vi "routine.vi"() -> ()   [LabVIEW 2011]
panel:
  in  "Boolean":bool
  in  "Filename":path=path "C:/Users/Sinha/Desktop/Ankle/2.csv"
  in  "Target":bool=TRUE
  in  "AI 2":bool
  in  "AI 1":bool=TRUE
  out "?":bool
  in  "AI 0":bool=TRUE
  in  "Target":dbl=0.5 caption="Offset"
  in  "Sample Rate Hz.":dbl=200.0
  out "Waveform Chart":dbl[][](graph)=[[-5.0, -5.0, -5.0, 0.5], [-5.0, -5.0, -5.0, 0.5], [-5.0, -5.0, -5.0, 0.5], [-5.0, -5.0, -5.0, 0.5], [-5.0, -5.0, -5.0, 0.5], [-5.0, -5.0, -5.0, 0.5], [-5.0, -5.0, -5.0, 0.5], [-5.0, -5.0, -5.0, 0.5], [-5.0, -5.0, -5.0, 0.5], [-5.0, -5.0, -5.0, 0.5], [-5.0, -5.0, -5.0, 0.5], [-5.0, -5.0, -5.0, 0.5], [-5.0, -5.0, -5.0, 0.5], [-5.0, -5.0, -5.0, 0.5], [-5.0, -5.0, -5.0, 0.5], [-5.0, -5.0, -5.0, 0.5], [-5.0, -5.0, -5.0, 0.5], [-5.0, -5.0, -5.0, 0.5], [-5.0, -5.0, -5.0, 0.5], [-5.0, -5.0, -5.0, 0.5]]
  in  "save":bool
  in  "stop (F)":bool caption="stop"
  # "USB"
  # "PCI"
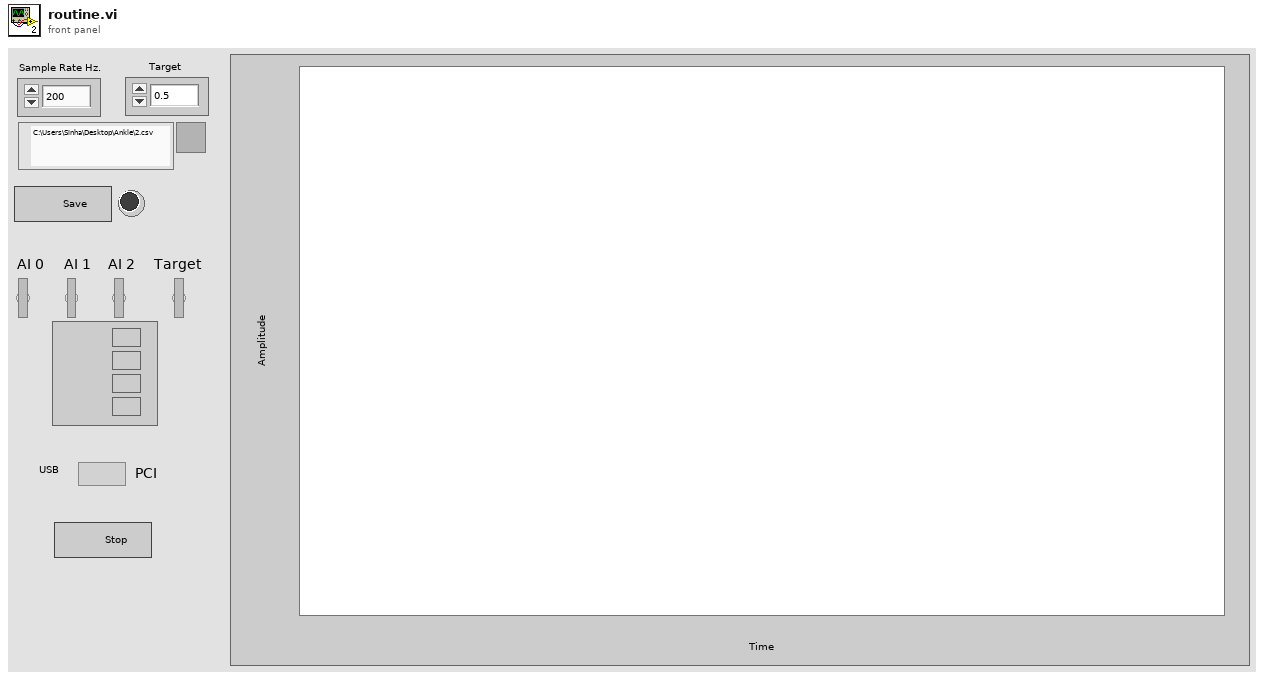
[diagram p1: front panel]
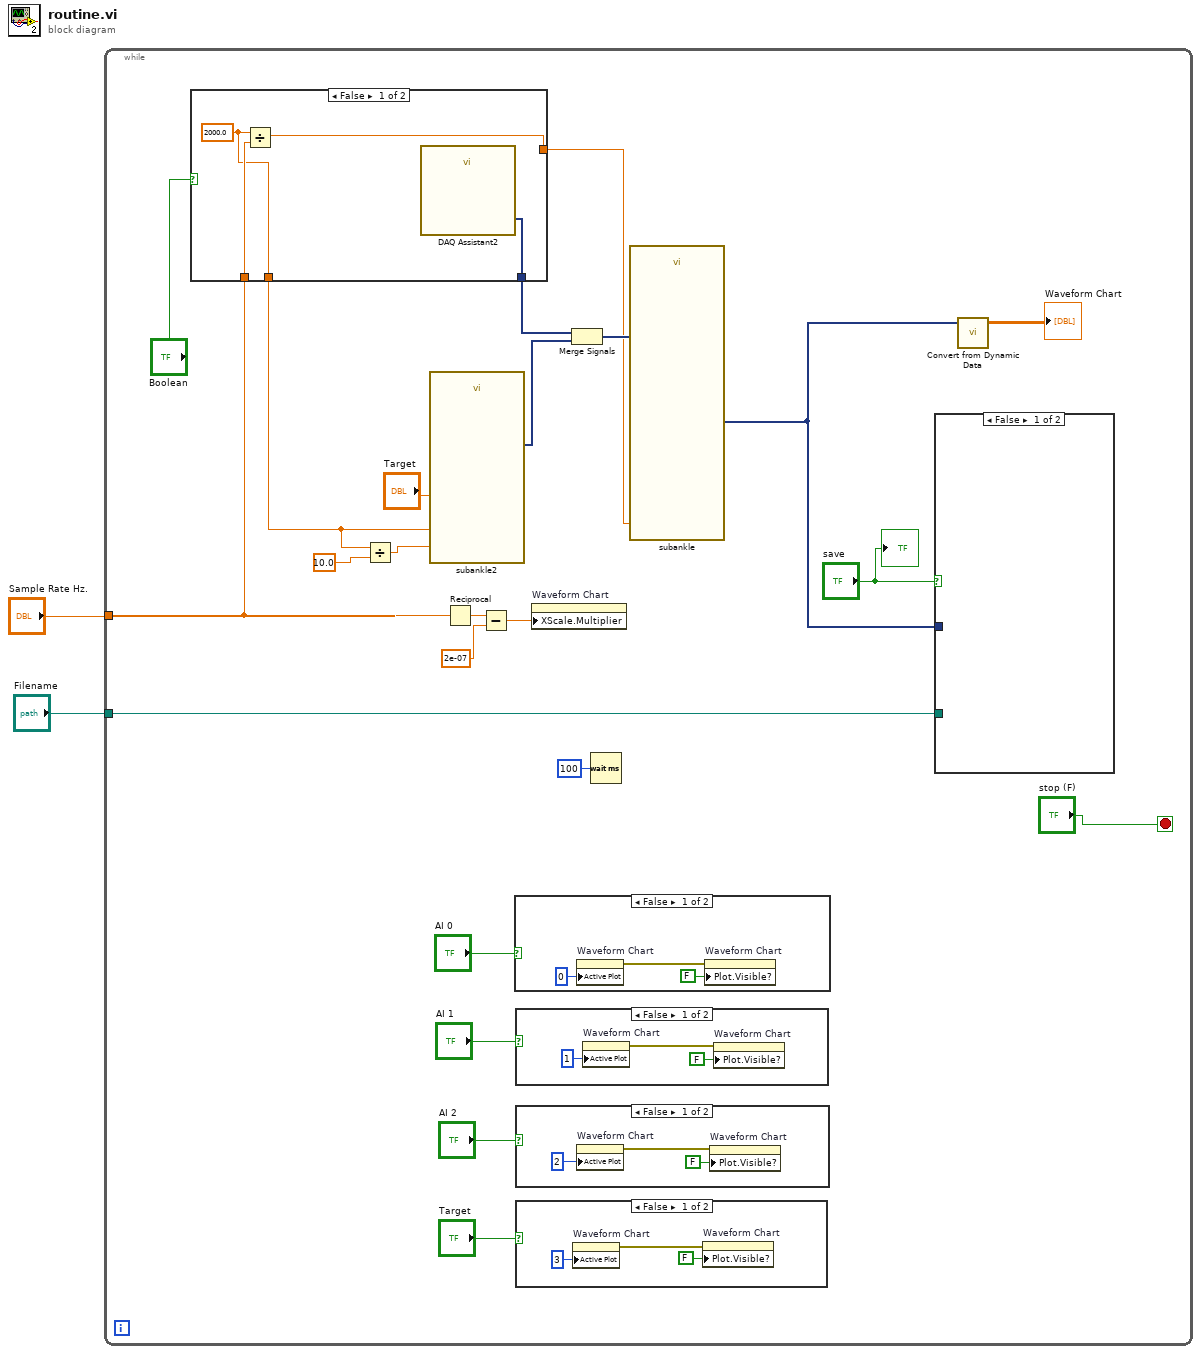
[diagram p0: block diagram]
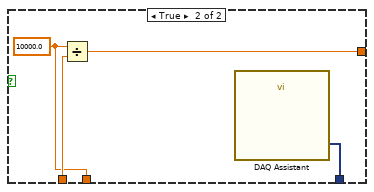
[diagram p2: hidden frame]
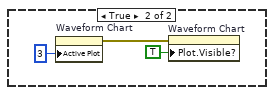
[diagram p3: hidden frame]
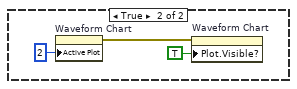
[diagram p4: hidden frame]
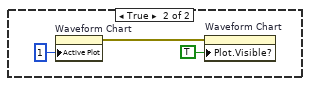
[diagram p5: hidden frame]
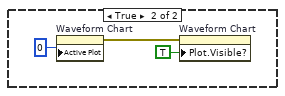
[diagram p6: hidden frame]
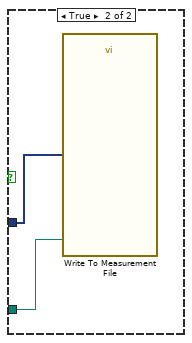
[diagram p7: hidden frame]
diagram:
  n1 = while {
    tunnel: "Sample Rate Hz." -> [w8]
    tunnel: "Filename" -> [w10]
    stop <- "stop (F)" stop-if-true
    n2 = case shown="False" "Boolean" {
      tunnel: [w29 w33] -> w19
      tunnel: w8 -> [w28 w32]
      tunnel: [w27 w31] -> w7
      tunnel: [w26 w30] -> w6
      frame False {
        w26 = 2000.0 ("x")
        n3 = Divide(x=w26, y=w28) -> (x/y=w27:dbl)
        n4 = call "DAQ Assistant2"() -> ("data"=w29:dynamicdata)  [unwired: 16 in, 3 out]
      }
      frame True {
        w30 = 10000.0 ("x")
        n5 = Divide(x=w30, y=w32) -> (x/y=w31:dbl)
        n6 = call "DAQ Assistant"() -> ("data"=w33:dynamicdata)  [unwired: 16 in, 3 out]
      }
    }
    n7 = Divide(x=w6, y=10.0) -> (x/y=w4:dbl)
    n8 = call "subankle2.vi"("Offset"="Target", "# of Samples"=w4, "Sampling Rate (Hz)"=w6) -> ("DC"=w18:dynamicdata)  [unwired: 11 in, 1 out]
    n9 = Reciprocal(x=w8) -> (1/x=w23:dbl)
    n10 = Subtract(x=w23, y=2e-07) -> (x-y=w21:dbl)
    n11 = case shown="False" "AI 0" {
      frame False {
        n12 = property on="Waveform Chart" class="WFChart (strict)"("Active Plot"=u32 0) -> (error out=w53:errorcluster)  [unwired: 2 in, 1 out]
        n13 = property on="Waveform Chart" class="WFChart (strict)"(error in=w53, "Plot.Visible?"=FALSE ("Plot.Visible")) -> ()  [unwired: 1 in, 2 out]
      }
      frame True {
        n14 = property on="Waveform Chart" class="WFChart (strict)"("Active Plot"=u32 0) -> (error out=w56:errorcluster)  [unwired: 2 in, 1 out]
        n15 = property on="Waveform Chart" class="WFChart (strict)"(error in=w56, "Plot.Visible?"=TRUE ("Plot.Visible")) -> ()  [unwired: 1 in, 2 out]
      }
    }
    n16 = case shown="False" "AI 1" {
      frame False {
        n17 = property on="Waveform Chart" class="WFChart (strict)"("Active Plot"=u32 1) -> (error out=w48:errorcluster)  [unwired: 2 in, 1 out]
        n18 = property on="Waveform Chart" class="WFChart (strict)"(error in=w48, "Plot.Visible?"=FALSE ("Plot.Visible")) -> ()  [unwired: 1 in, 2 out]
      }
      frame True {
        n19 = property on="Waveform Chart" class="WFChart (strict)"("Active Plot"=u32 1) -> (error out=w51:errorcluster)  [unwired: 2 in, 1 out]
        n20 = property on="Waveform Chart" class="WFChart (strict)"(error in=w51, "Plot.Visible?"=TRUE ("Plot.Visible")) -> ()  [unwired: 1 in, 2 out]
      }
    }
    n21 = case shown="False" "AI 2" {
      frame False {
        n22 = property on="Waveform Chart" class="WFChart (strict)"("Active Plot"=u32 2) -> (error out=w42:errorcluster)  [unwired: 2 in, 1 out]
        n23 = property on="Waveform Chart" class="WFChart (strict)"(error in=w42, "Plot.Visible?"=FALSE ("Plot.Visible")) -> ()  [unwired: 1 in, 2 out]
      }
      frame True {
        n24 = property on="Waveform Chart" class="WFChart (strict)"("Active Plot"=u32 2) -> (error out=w44:errorcluster)  [unwired: 2 in, 1 out]
        n25 = property on="Waveform Chart" class="WFChart (strict)"(error in=w44, "Plot.Visible?"=TRUE ("Plot.Visible")) -> ()  [unwired: 1 in, 2 out]
      }
    }
    n26 = case shown="False" "Target" {
      frame False {
        n27 = property on="Waveform Chart" class="WFChart (strict)"("Active Plot"=u32 3) -> (error out=w36:errorcluster)  [unwired: 2 in, 1 out]
        n28 = property on="Waveform Chart" class="WFChart (strict)"(error in=w36, "Plot.Visible?"=FALSE ("Plot.Visible")) -> ()  [unwired: 1 in, 2 out]
      }
      frame True {
        n29 = property on="Waveform Chart" class="WFChart (strict)"("Active Plot"=u32 3) -> (error out=w38:errorcluster)  [unwired: 2 in, 1 out]
        n30 = property on="Waveform Chart" class="WFChart (strict)"(error in=w38, "Plot.Visible?"=TRUE ("Plot.Visible")) -> ()  [unwired: 1 in, 2 out]
      }
    }
    n31 = property on="Waveform Chart" class="WFChart (strict)"("XScale.Multiplier"=w21) -> ()  [unwired: 2 in, 2 out]
    n32 = Merge Signals(w19, w18) -> (w17:dynamicdata)
    n33 = Wait (ms)(milliseconds to wait=u32 100) -> ()  [unwired: 1 out]
    n34 = call "subankle.vi"("Size"=w7, "Signals"=w17) -> ("Median"=w3:dynamicdata)  [unwired: 3 in, 6 out]
    n35 = case shown="False" "save" {
      tunnel: w3 -> [_ w58]
      tunnel: w10 -> [_ w59]
      frame False {
      }
      frame True {
        n36 = call "Write To Measurement File"("Signals"=w58, "Filename"=w59) -> ()  [unwired: 15 in, 3 out]
      }
    }
    n37 = call "Convert from Dynamic Data"("Dynamic Data Type"=w3) -> ("Array"=→"Waveform Chart":dbl[][])  [unwired: 3 in]
    "?" <- "save"
  }
